vi "MegaAwesome_8_28_12b_JW.vi"() -> ()   [LabVIEW 2011]
uses:
  MegaAwesome_States.ctl
panel:
  out "Sat Id-Used":dbl[](array[numeric])
  out "Sat Vg Array-Used":dbl[](array[numeric])
  out "Vg Array-Log-Used":dbl[](array[numeric])
  out "Sat Id-Log-Used":dbl[](array[numeric])
  out "Lin Id-Used":dbl[](array[numeric])
  out "Lin-Vg Array-Used":dbl[](array[numeric])
  out "Lin Vd":dbl
  out "Recorded Prop":T1
  in  "Room Temp":dbl=294.0
  out "Current State":T2
  in  "Main Tab Control":T3(tab)
  in  "Image Folder":path
  out "Image File":path=path "D:/UserData/Desktop/Jeremy/WFU/Research/Programs/VI mods/Image Not Found.png"
  in  "Transfer File":path
  out "Transfer Folder":path
  out "Fabrication Prop":T4
  out "Image Preview":T5(plugin-control)
  out "Image Out":T5(plugin-control)
  out "Image Name":string
  out "Index":string
  out "Date Created":string caption="Fabricated"
  in  "Comments:":string
  out "Rec: Length":dbl caption="Length" format="%#_3g"
  out "Rec: Width":dbl caption="Width" format="%#_4g"
  out "Rec: Dielectric (d)":dbl caption="Dielectric (d)" format="%#_3g"
  in  "New: Dielectric":dbl
  in  "New: Length":dbl
  in  "New: Width":dbl
  out "Rec: Temp":dbl caption="Sample Temp" format="%.1f"
  in  "New: Temp":dbl format="%.1f"
  in  "Num Pts":dbl=5.0
  in  "Num Pts Log":dbl=5.0 caption="Num Pts"
  out "Recorded Values Cluster":T6
  out "Calculated Values Cluster":T6 caption="Recorded Values Cluster"
  out "Re-Calculated Values Cluster":T6 caption="Recorded Values Cluster"
  in  "Origin Project File":path=path "\\\\acad1\\physics/Jurchescu-group/JW-PD/Group Library/Origin Project Files/DeviceData_8_10_12a_JW.opj"
  in  "No Image File":path=path "\\\\acad1\\physics/Jurchescu-group/JW-PD/Mega Awesome/Image Not Found.png"
  # "Image Location"
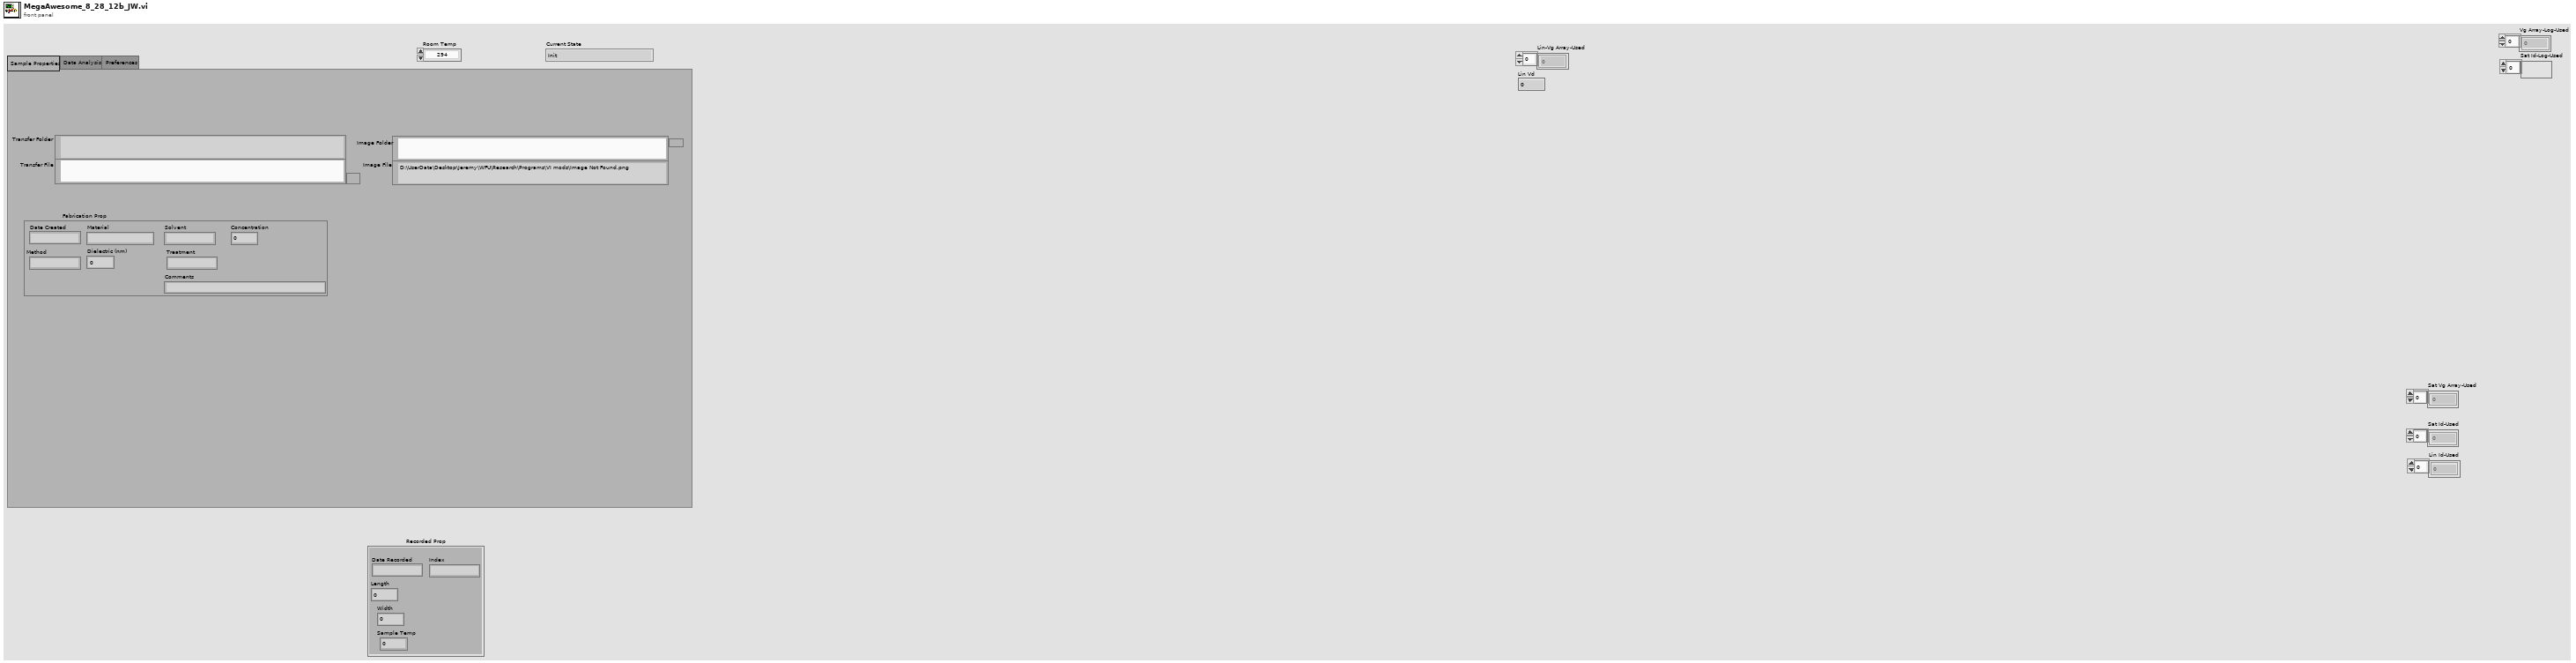
[diagram p1: front panel]
types:
  T1 = cluster{"Date Recorded":string, "Index":string, "Length":dbl, "Width":dbl, "Sample Temp":dbl}
  T2 = typedef "MegaAwesome_States.ctl" = enum16{"Init", "File Missing", "No Event", "Read Data", "Calculated Values", "Re-Calculated Values", "Exit"}
  T3 = enum32{"Sample Properties", "Data Analysis", "Preferences"}
  T4 = cluster{"Date Created":string, "Material":string, "Solvent":string, "Concentration":dbl, "Method":string, "Dielectric (nm)":dbl, "Treatment":string, "Comments":string}
  T5 = typedef "IMAQ Image.ctl" = refnum<image>
  T6 = cluster{"Mobility-Sat":dbl, "Moblitity-Lin":dbl, "On/Off":dbl, "Off Current":dbl, "Vt-Sat":dbl, "STS":dbl, "Trap Density-VT":dbl, "Trap Density-STS":dbl}
  T7 = cluster{"Mobility-Sat":dbl, "Vt-Sat":dbl, "Mobility-Lin":dbl, "Vt-Lin":dbl, "Off I-Sat":dbl, "On/Off I-Sat":dbl}
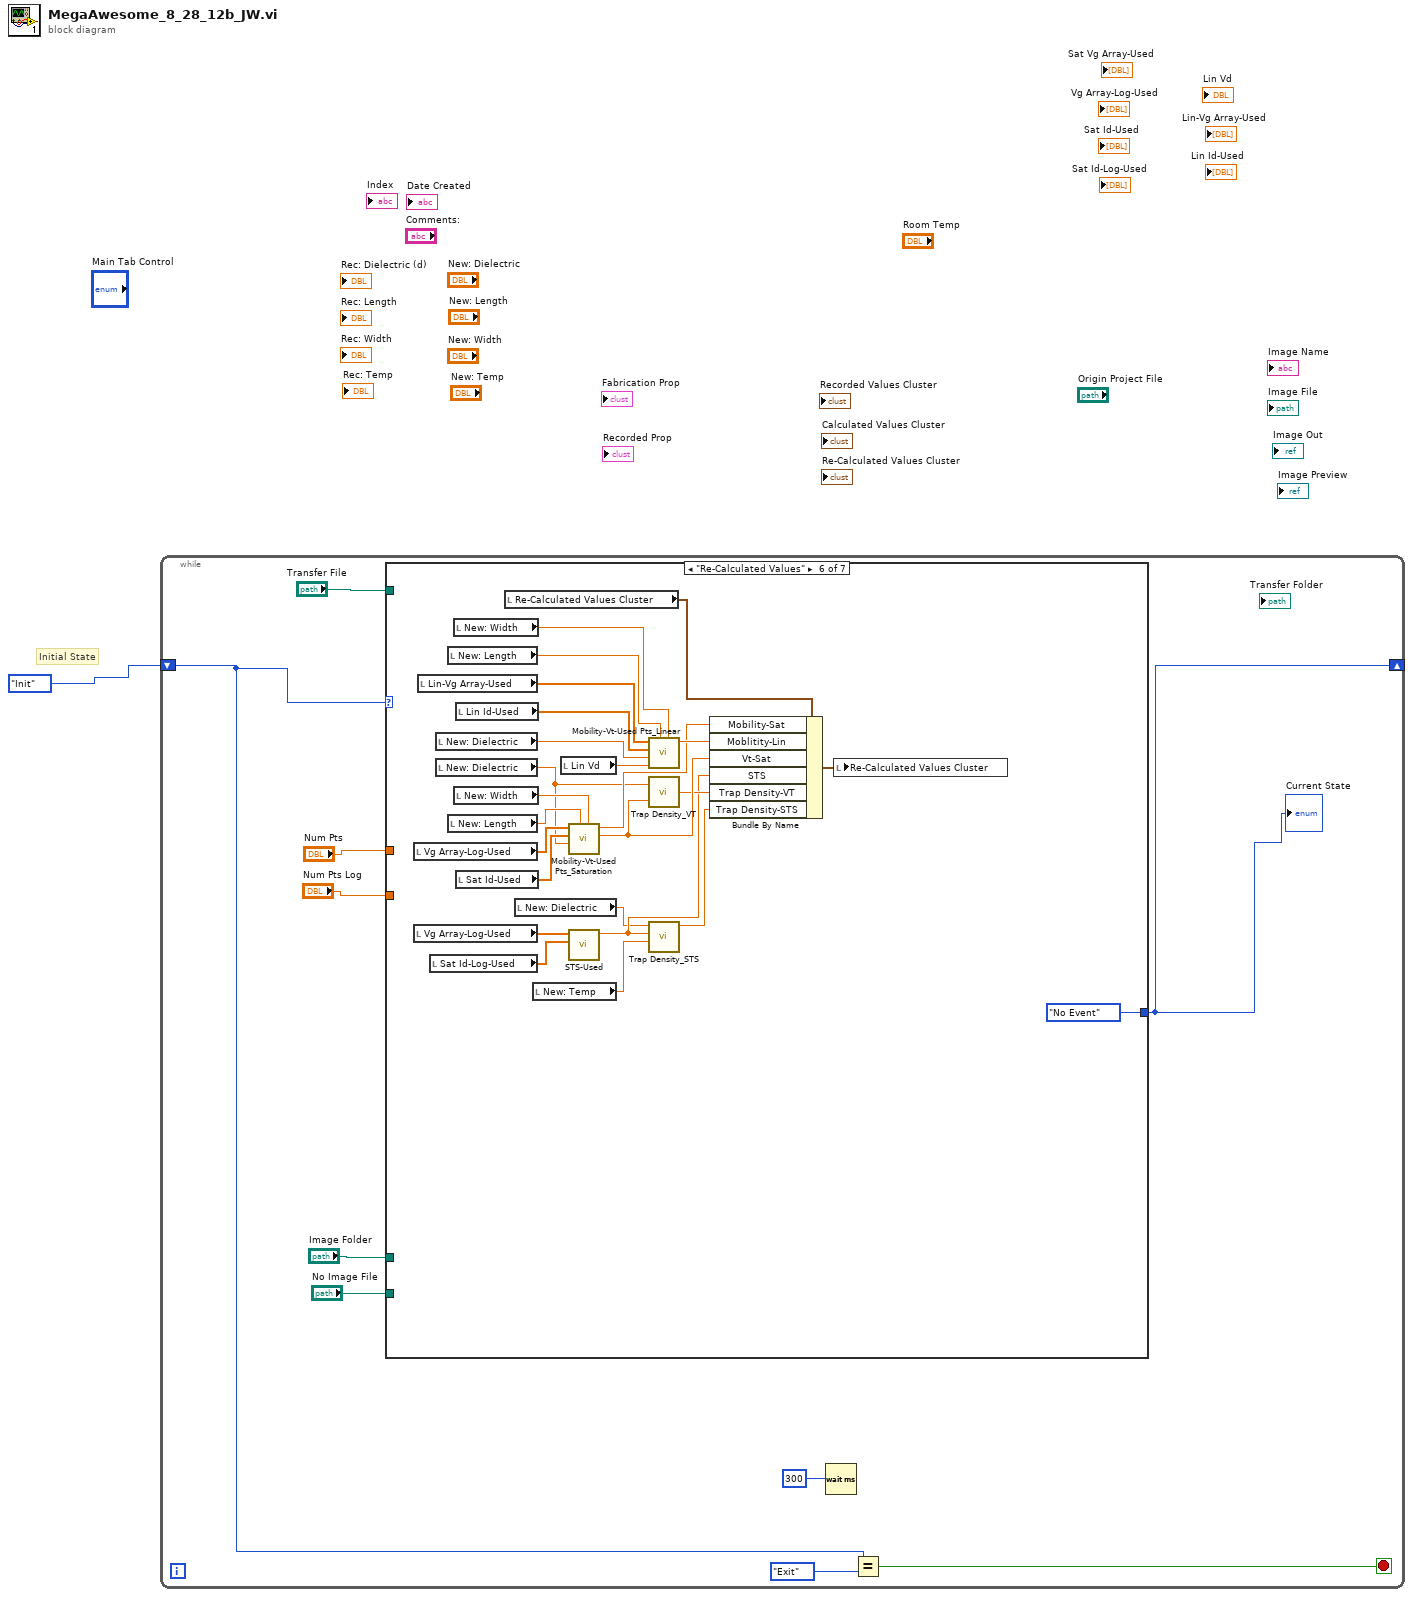
[diagram p0: block diagram]
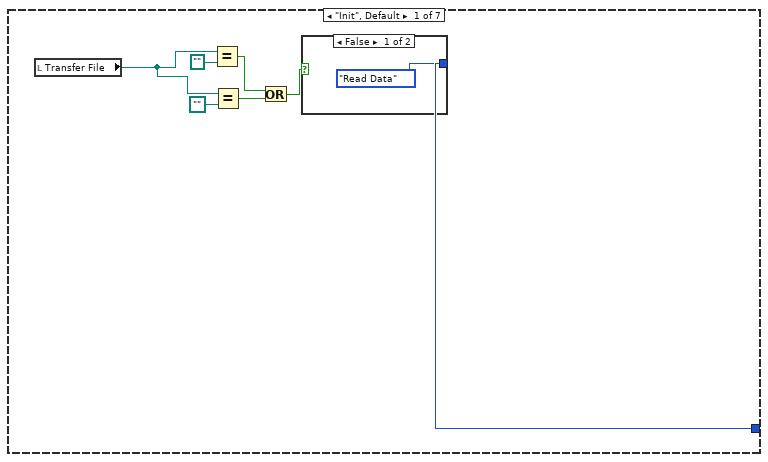
[diagram p2: hidden frame]
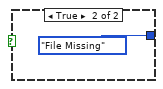
[diagram p3: hidden frame]
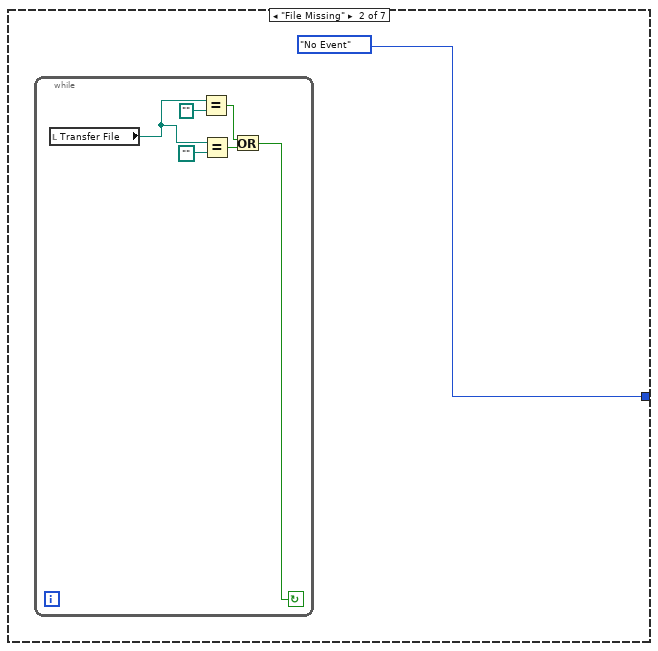
[diagram p4: hidden frame]
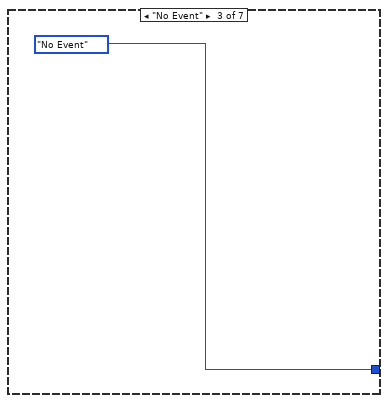
[diagram p5: hidden frame]
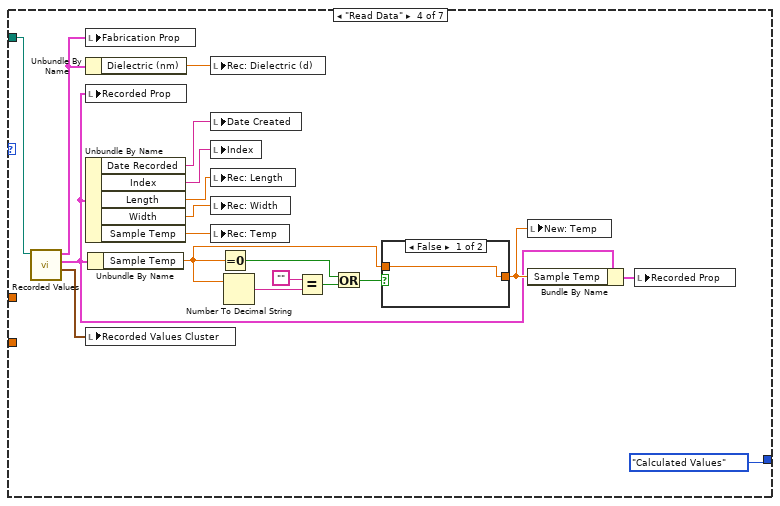
[diagram p6: hidden frame]
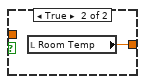
[diagram p7: hidden frame]
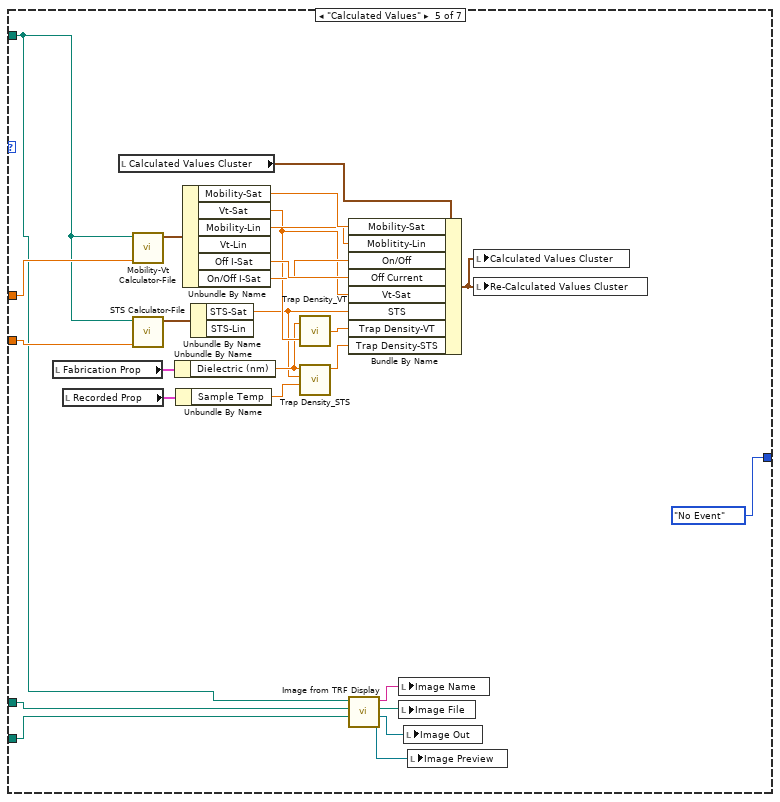
[diagram p8: hidden frame]
diagram:
  # "Initial State"
  n1 = while {
    shift-right: [w7] -> _
    shift-left: MegaAwesome_States."Init" -> [w10]
    stop <- w11 stop-if-true
    n2 = case shown="\"Re-Calculated Values\"" w10 {
      selector: w10 -> [_ _ _ _ _ _ w100]
      tunnel: [w12 MegaAwesome_States."No Event" MegaAwesome_States."No Event" MegaAwesome_States."Calculated Values" MegaAwesome_States."No Event" MegaAwesome_States."No Event" w100] -> w7
      tunnel: "Transfer File" -> [_ _ _ w47 w56 _ _]
      tunnel: "Num Pts" -> [_ _ _ _ w60 _ _]
      tunnel: "Num Pts Log" -> [_ _ _ _ w59 _ _]
      tunnel: "Image Folder" -> [_ _ _ _ w55 _ _]
      tunnel: "No Image File" -> [_ _ _ _ w54 _ _]
      frame "Init", Default {
        n3 = local read "Transfer File"() -> (w13:path)
        n4 = Equal?(x=w13, y=path "") -> (x = y?=w16:bool)
        n5 = Equal?(x=w13, y=path "") -> (x = y?=w15:bool)
        n6 = Or(x=w16, y=w15) -> (x .or. y?=w18:bool)
        n7 = case shown="False" w18 {
          tunnel: [MegaAwesome_States."Read Data" MegaAwesome_States."File Missing"] -> w12
          frame False {
          }
          frame True {
          }
        }
      }
      frame "File Missing" {
        n8 = while {
          stop <- w22 continue-if-true
          n9 = local read "Transfer File"() -> (w23:path)
          n10 = Equal?(x=w23, y=path "") -> (x = y?=w25:bool)
          n11 = Equal?(x=w23, y=path "") -> (x = y?=w26:bool)
          n12 = Or(x=w25, y=w26) -> (x .or. y?=w22:bool)
        }
      }
      frame "No Event" {
      }
      frame "Read Data" {
        n13 = call "Recorded Values.vi"("Path"=w47) -> ("Recorded Char"=w46:T6, "Recorded Prop"=w36:T1, "Fabrication Prop"=w30:T4)  [unwired: 8 in]
        n14 = local write "Fabrication Prop"(w30) -> ()
        n15 = Unbundle By Name(w30) -> ("Dielectric (nm)"=w29:dbl)
        n16 = local write "Recorded Prop"(w36) -> ()
        n17 = Unbundle By Name(w36) -> ("Date Recorded"=w35:string, "Index"=w33:string, "Length"=w34:dbl, "Width"=w32:dbl, "Sample Temp"=w31:dbl)
        n18 = local write "Recorded Values Cluster"(w46) -> ()
        n19 = Unbundle By Name(w36) -> ("Sample Temp"=w39:dbl)
        n20 = local write "Rec: Dielectric (d)"(w29) -> ()
        n21 = local write "Date Created"(w35) -> ()
        n22 = local write "Index"(w33) -> ()
        n23 = local write "Rec: Length"(w34) -> ()
        n24 = local write "Rec: Width"(w32) -> ()
        n25 = local write "Rec: Temp"(w31) -> ()
        n26 = Equal To 0?(x=w39) -> (x = 0?=w42:bool)
        n27 = Number To Decimal String(number=w39) -> (decimal integer string=w43:string)  [unwired: 1 in]
        n28 = Equal?(x="", y=w43) -> (x = y?=w41:bool)
        n29 = Or(x=w42, y=w41) -> (x .or. y?=w40:bool)
        n30 = case shown="False" w40 {
          tunnel: [w48 w49] -> w37
          tunnel: w39 -> [w48 _]
          frame False {
          }
          frame True {
            n31 = local read "Room Temp"() -> (w49:dbl)
          }
        }
        n32 = local write "New: Temp"(w37) -> ()
        n33 = Bundle By Name(cluster=w36, "Sample Temp"=w37) -> (w38:T1)
        n34 = local write "Recorded Prop"(w38) -> ()
      }
      frame "Calculated Values" {
        n35 = local read "Fabrication Prop"() -> (w65:T4)
        n36 = local read "Recorded Prop"() -> (w58:T1)
        n37 = local read "Calculated Values Cluster"() -> (w75:T6)
        n38 = call "Mobility-Vt Calculator-File.vi"("NumPts"=w60, "Path"=w56) -> ("Output"=w73:T7)  [unwired: 5 in, 4 out]
        n39 = call "STS Calculator-File.vi"("NumPts"=w59, "Path"=w56) -> ("Ouput"=w68:cluster{"STS-Sat":dbl, "STS-Lin":dbl})  [unwired: 5 in, 4 out]
        n40 = Unbundle By Name(w65) -> ("Dielectric (nm)"=w63:dbl)
        n41 = Unbundle By Name(w58) -> ("Sample Temp"=w57:dbl)
        n42 = Unbundle By Name(w73) -> ("Mobility-Sat"=w72:dbl, "Vt-Sat"=w64:dbl, "Mobility-Lin"=w71:dbl, "Off I-Sat"=w70:dbl, "On/Off I-Sat"=w69:dbl)  [unwired: 1 out]
        n43 = Unbundle By Name(w68) -> ("STS-Sat"=w62:dbl)  [unwired: 1 out]
        n44 = call "Trap Density_VT.vi"("VT"=w64, "Dielectric"=w63) -> ("Trap Density-VT"=w67:dbl)
        n45 = call "Trap Density_STS.vi"("Temp (T) [K]"=w57, "S.T.S. (S)"=w62, "Dielectric"=w63) -> ("Trap Density (N)"=w66:dbl)  [unwired: 8 in]
        n46 = Bundle By Name(cluster=w75, "Mobility-Sat"=w72, "Moblitity-Lin"=w71, "On/Off"=w69, "Off Current"=w70, "Vt-Sat"=w64, "STS"=w62, "Trap Density-VT"=w67, "Trap Density-STS"=w66) -> (w74:T6)
        n47 = call "Image from TRF Display.vi"("No Image File"=w54, "Image Folder"=w55, "Transfer File"=w56) -> ("Image Out 2"=w50:T5, "Image Out"=w51:T5, "Image File"=w52:path, "Image Name"=w53:string)  [unwired: 5 in]
        n48 = local write "Image Name"(w53) -> ()
        n49 = local write "Image File"(w52) -> ()
        n50 = local write "Image Out"(w51) -> ()
        n51 = local write "Image Preview"(w50) -> ()
        n52 = local write "Calculated Values Cluster"(w74) -> ()
        n53 = local write "Re-Calculated Values Cluster"(w74) -> ()
      }
      frame "Re-Calculated Values" {
        n54 = local read "Vg Array-Log-Used"() -> (w90:dbl[])
        n55 = local read "Vg Array-Log-Used"() -> (w82:dbl[])
        n56 = local read "Lin-Vg Array-Used"() -> (w97:dbl[])
        n57 = local read "Sat Id-Log-Used"() -> (w81:dbl[])
        n58 = local read "New: Dielectric"() -> (w95:dbl)
        n59 = local read "New: Dielectric"() -> (w79:dbl)
        n60 = local read "New: Length"() -> (w93:dbl)
        n61 = local read "New: Length"() -> (w89:dbl)
        n62 = local read "New: Width"() -> (w92:dbl)
        n63 = local read "New: Width"() -> (w88:dbl)
        n64 = local read "Lin Id-Used"() -> (w96:dbl[])
        n65 = local read "Sat Id-Used"() -> (w87:dbl[])
        n66 = local read "Re-Calculated Values Cluster"() -> (w99:T6)
        n67 = local read "New: Dielectric"() -> (w78:dbl)
        n68 = local read "New: Temp"() -> (w77:dbl)
        n69 = local read "Lin Vd"() -> (w94:dbl)
        n70 = call "Mobility-Vt-Used Pts_Saturation.vi"("Width"=w88, "Length"=w89, "Dielectric (d)"=w79, "Sat Id Used"=w87, "Vg Used"=w90) -> ("Vt"=w85:dbl, "Mobility"=w86:dbl)  [unwired: 4 in, 1 out]
        n71 = call "STS-Used.vi"("Id Used"=w81, "Vg-Used"=w82) -> ("STS"=w80:dbl)  [unwired: 9 in]
        n72 = call "Mobility-Vt-Used Pts_Linear.vi"("Width"=w92, "Length"=w93, "Vd"=w94, "Dielectric (d)"=w95, "Sat Id Used"=w96, "Vg Used"=w97) -> ("Mobility"=w91:dbl)  [unwired: 3 in, 2 out]
        n73 = call "Trap Density_VT.vi"("VT"=w85, "Dielectric"=w79) -> ("Trap Density-VT"=w84:dbl)
        n74 = call "Trap Density_STS.vi"("Temp (T) [K]"=w77, "S.T.S. (S)"=w80, "Dielectric"=w78) -> ("Trap Density (N)"=w76:dbl)  [unwired: 8 in]
        n75 = Bundle By Name(cluster=w99, "Mobility-Sat"=w86, "Moblitity-Lin"=w91, "Vt-Sat"=w85, "STS"=w80, "Trap Density-VT"=w84, "Trap Density-STS"=w76) -> (w98:T6)
        n76 = local write "Re-Calculated Values Cluster"(w98) -> ()
      }
      frame "Exit" {
      }
    }
    "Current State" <- w7
    n77 = Wait (ms)(milliseconds to wait=300) -> ()  [unwired: 1 out]
    n78 = Equal?(x=w10, y=MegaAwesome_States."Exit") -> (x = y?=w11:bool)
  }
